vi "test Diff Configuration (Add Remove RTs).vi"(8 "error in":errorcluster, 11 "TestCase in":refnum<class "Refresh.lvclass">) -> (0 "error out":errorcluster, 3 "TestCase out":refnum<class "Refresh.lvclass">)   [LabVIEW 2020, in "Refresh.lvclass"]
uses:
  Refresh.lvclass
  <vilib>/addons/_JKI Toolkits/VI Tester/TestCase.llb/TestCase.lvclass
  System Explorer/Implementation/System Explorer/Refresh/Refresh.lvlib
  Shared/Parameter Definition.ctl
  Shared/Address.ctl
  Shared/Terminal Endpoint.ctl
  Shared/Message Type.ctl
  Shared/Message Definition.ctl
  Shared/1553 Channel.ctl
  System Explorer/Implementation/System Explorer/Refresh/Symbols.ctl
  System Explorer/Implementation/System Explorer/Refresh/Change Type.ctl
  System Explorer/Implementation/System Explorer/Refresh/MCL Row.ctl
  C:/Program Files (x86)/National Instruments/LabVIEW 2020/vi.lib/addons/_JKI Toolkits/VI Tester/TestCase.llb/TestCase.lvclass
panel:
  out "Multicolumn Listbox":i32(listbox)=-1
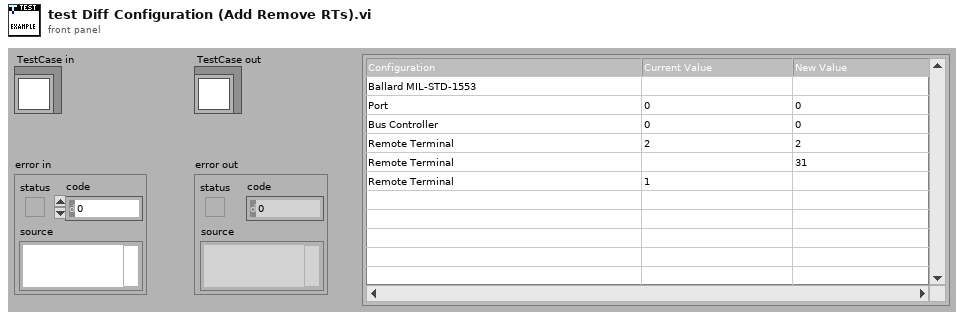
[diagram p1: front panel]
types:
  T1 = typedef "Address.ctl" = u16
  T2 = typedef "1553 Channel.ctl" = cluster{"HW channel":u16, "terminal addresses":T1[], "acyclic frame names":string[], "messages":T3[]}
  T3 = typedef "Message Definition.ctl" = cluster{"name":string, "message type":T4, "endpoint Rx":T5, "endpoint Tx":T5, "mode code":u16, "number of words":u16, "parameters":cluster{"name":string, "default value":dbl, "unit":string, "parameter definition":T6}[], "create timestamp channel":bool}
  T4 = typedef "Message Type.ctl" = string
  T5 = typedef "Terminal Endpoint.ctl" = cluster{"terminal address":T1, "subaddress":T1}
  T6 = typedef "Parameter Definition.ctl" = cluster{"start index":i32, "size (bits)":i32, "encoding":enum16{"BNR", "BCD", "Discrete"}, "signed":bool, "multiplier":dbl, "offset":dbl}
  T7 = typedef "Ballard MIL-STD-1553 System Explorer.lvlib/Implementation.lvlib/Refresh.lvlib/MCL Row.ctl" = cluster{"change type":T8, "item symbol":T9, "item names":string[]}
  T8 = typedef "Ballard MIL-STD-1553 System Explorer.lvlib/Implementation.lvlib/Refresh.lvlib/Change Type.ctl" = enum16{"No change", "Modify", "Add", "Remove"}
  T9 = typedef "Ballard MIL-STD-1553 System Explorer.lvlib/Implementation.lvlib/Refresh.lvlib/Symbols.ctl" = enum16{"Blank", "MIL-STD-1553", "Port", "Remote Terminal", "Subaddress", "Bus Controller", "Acyclic Frame", "Mode Code", "Message", "Parameter", "Item"}
  T10 = typedef "imagedata.ctl" = cluster{"image type":i32, "image depth":i32, "image":u8[], "mask":u8[], "colors":u32[], "Rectangle":cluster{"left":i16, "top":i16, "right":i16, "bottom":i16}}
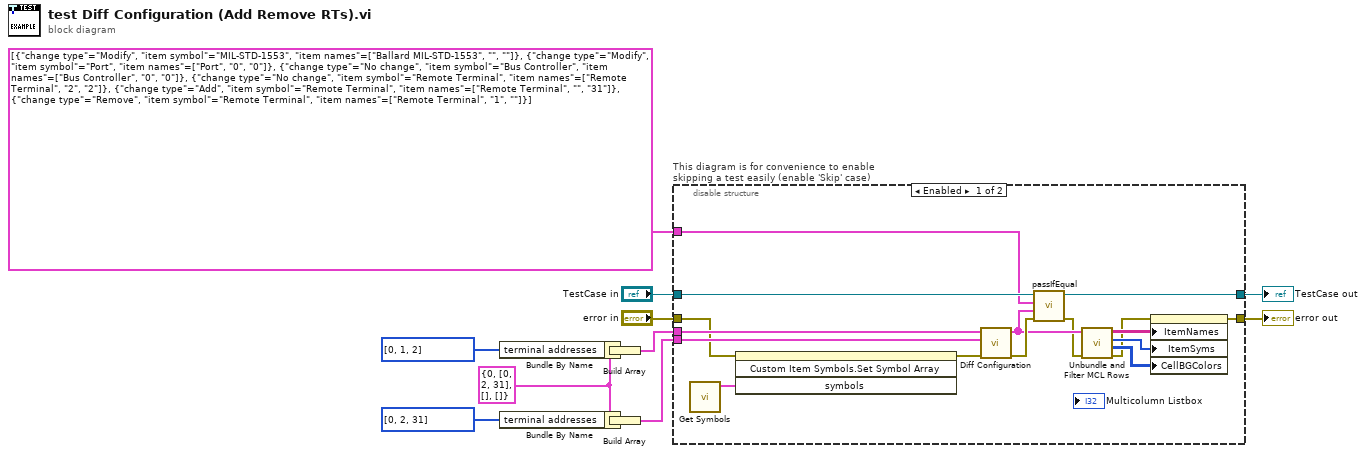
[diagram p0: block diagram]
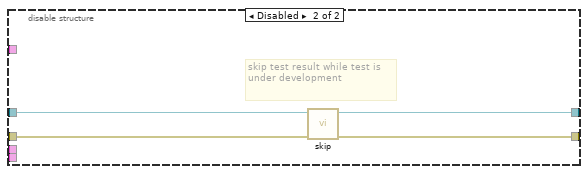
[diagram p2: hidden frame]
diagram:
  w5 = T2 {"HW channel"=0, "terminal addresses"=[0, 2, 31], "acyclic frame names"=[], "messages"=[]} ("1553 channel")
  n1 = Bundle By Name(cluster=w5, "terminal addresses"=T1[] [0, 1, 2] ("terminals")) -> (w4:T2)
  n2 = Bundle By Name(cluster=w5, "terminal addresses"=T1[] [0, 2, 31] ("terminals")) -> (w2:T2)
  n3 = Build Array(w4) -> (w3:T2[])
  n4 = Build Array(w2) -> (w1:T2[])
  n5 = disable-structure "This diagram is for convenience to enable skipping a test easily (enable 'Skip' case)" shown="Enabled" {
    disable-tunnel: "TestCase in" -> [w28 w32]
    disable-tunnel: [w27 w30] -> w9
    disable-tunnel: [w16 w31] -> w11
    disable-tunnel: "error in" -> [w14 w29]
    disable-tunnel: w3 -> [w26 _]
    disable-tunnel: w1 -> [w25 _]
    disable-tunnel: T7[] [{"change type"=enum."Modify", "item symbol"=enum."MIL-STD-1553", "item names"=["Ballard MIL-STD-1553", "", ""]}, {"change type"=enum."Modify", "item symbol"=enum."Port", "item names"=["Port", "0", "0"]}, {"change type"=enum."No change", "item symbol"=enum."Bus Controller", "item names"=["Bus Controller", "0", "0"]}, {"change type"=enum."No change", "item symbol"=enum."Remote Terminal", "item names"=["Remote Terminal", "2", "2"]}, {"change type"=enum."Add", "item symbol"=enum."Remote Terminal", "item names"=["Remote Terminal", "", "31"]}, {"change type"=enum."Remove", "item symbol"=enum."Remote Terminal", "item names"=["Remote Terminal", "1", ""]}] ("configuration diff") -> [w24 _]
    frame Enabled {
      n6 = call "Get Symbols.vi"() -> ("MIL-STD-1553 symbols"=w15:T10[])  [unwired: 11 in]
      n7 = invoke on="Multicolumn Listbox" class="MCListbox (strict)" method="Custom Item Symbols.Set Symbol Array"(error in=w14, "symbols"=w15) -> (error out=w13:errorcluster)  [unwired: 2 in, 3 out]
      n8 = call "Diff Configuration.vi"("error in"=w13, "configuration new"=w25, "configuration old"=w26) -> ("error out"=w23:errorcluster, "configuration diff"=w22:T7[])  [unwired: 7 in]
      n9 = call-dynamic "passIfEqual.vi"("error in (no error)"=w23, "y"=w22, "x"=w24, "TestCase in"=w28) -> ("error out"=w18:errorcluster, "TestCase out"=w27:refnum<class "Refresh.lvclass">)  [unwired: 6 in]
      n10 = call "Unbundle and Filter MCL Rows.vi"("error in"=w18, "refresh items"=w22) -> ("error out"=w17:errorcluster, "background colors"=w21:u32[][], "item symbols"=w20:T9[], "item names"=w19:string[][])  [unwired: 6 in]
      n11 = property on="Multicolumn Listbox" class="MCListbox (strict)"(error in=w17, "ItemNames"=w19, "ItemSyms"=w20, "CellBGColors"=w21) -> (error out=w16:errorcluster)  [unwired: 1 in, 1 out]
    }
    frame Disabled {
      # "skip test result while test is under development"
      n12 = call <vilib>:"skip.vi"("error in (no error)"=w29, "TestCase in"=w32) -> ("error out"=w31:errorcluster, "TestCase out"=w30:refnum<class "Refresh.lvclass">)  [unwired: 8 in]
    }
  }
  "error out" <- w11
  "TestCase out" <- w9
